vi "SQL_monitor_data_settinngs_select.vi"() -> (0 "报警级别设置":string[][](table), 1 "error out":errorcluster, 3 "工作条件及报警门限参考值设定":string[][](table))   [LabVIEW 2014]
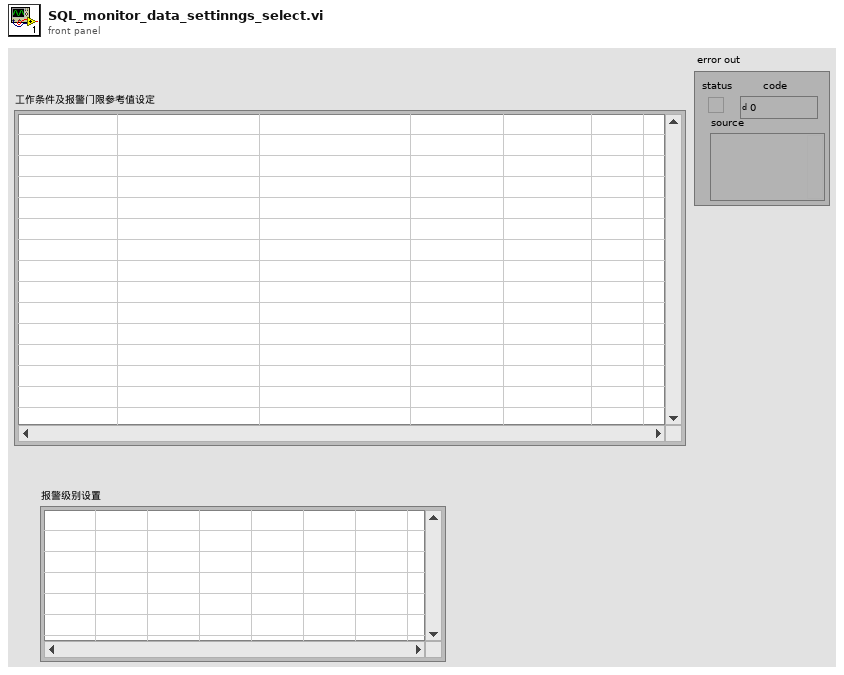
[diagram p1: front panel]
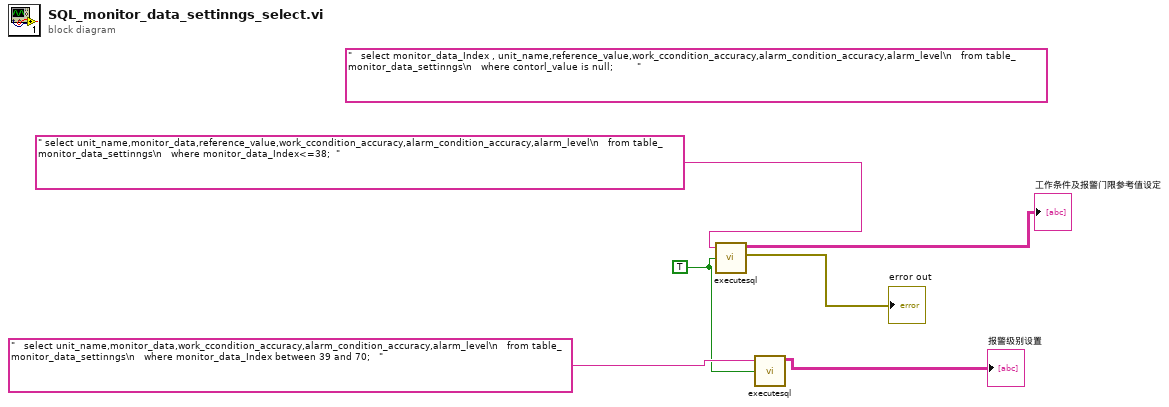
[diagram p0: block diagram]
diagram:
  w3 = TRUE
  (unwired) "   select monitor_data_Index , unit_name,reference_value,work_ccondition_accuracy,alarm_condition_accuracy,alarm_level\n   from table_monitor_data_settinngs\n   where contorl_value is null;        "
  n1 = call "executesql.vi"("Return Data (T)"=w3, "Command Text"=" select unit_name,monitor_data,reference_value,work_ccondition_accuracy,alarm_condition_accuracy,alarm_level\n   from table_monitor_data_settinngs\n   where monitor_data_Index<=38;  ") -> ("error out"=→"error out":errorcluster, "Data"=→"工作条件及报警门限参考值设定":string[][])  [unwired: 5 in]
  n2 = call "executesql.vi"("Return Data (T)"=w3, "Command Text"="   select unit_name,monitor_data,work_ccondition_accuracy,alarm_condition_accuracy,alarm_level\n   from table_monitor_data_settinngs\n   where monitor_data_Index between 39 and 70;   ") -> ("Data"=→"报警级别设置":string[][])  [unwired: 5 in, 1 out]
